vi "Module Cleanup.vi"(8 "error in (no error)":errorcluster, 11 "Messaging Client in":refnum<class "Messaging Server Client.lvclass">) -> (0 "error out":errorcluster, 3 "Messaging Client out":refnum<class "Messaging Server Client.lvclass">)   [LabVIEW 2020, in "Volatus.lvlib" / "Messaging Server Client.lvclass"]
uses:
  Messaging Server Client.lvclass
  Messaging Server Client.lvclass/Messaging Server Client.ctl
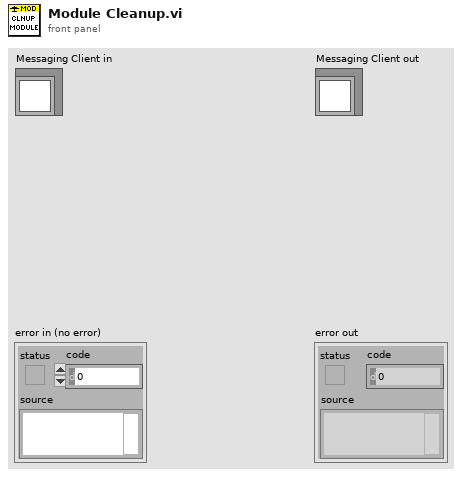
[diagram p1: front panel]
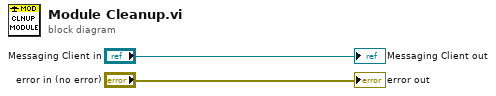
[diagram p0: block diagram]
diagram:
  "error out" <- "error in (no error)"
  "Messaging Client out" <- "Messaging Client in"
